vi "JoystickToPWMScale.vi"(10 "Numeric":i16) -> (2 "Numeric 2":u16)   [LabVIEW 2013, in "ProcessorHelperFunctions.lvlib"]
uses:
  ProcessorHelperFunctions.lvlib
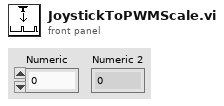
[diagram p1: front panel]
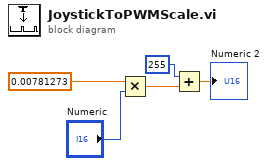
[diagram p0: block diagram]
diagram:
  n1 = Multiply(x=0.00781273, y="Numeric") -> (x*y=w4:dbl)
  n2 = Add(x=255, y=w4) -> (x+y=→"Numeric 2":dbl)
